vi "Asylum_Driver.vi"() -> ()   [LabVIEW 2019]
uses:
  subVIs/AFM API/AFM_Driver_Manager/AFM_Driver_Manager.PublicEvents.ctl
  subVIs/AFM API/AFM_Driver_Manager/AFM_Driver_Manager.PublicMethods.ctl
  <userlib>/LevyLab/Relay Box/Typedefs/Resistor--enum.ctl
  <userlib>/LevyLab/Configuration/Configuration.lvclass
  Type Defs/Asylum Configuration.ctl
  <vilib>/Utility/sysdir.llb/Get System Directory.vi
  <userlib>/LevyLab/Relay Box/Relay-Box.lvclass
  subVIs/AFM API/AFM_Driver_Manager/AFM_Driver_Manager.lvclass
panel:
  out "Debug Mode?":bool
  in  "Writing Setpoint":dbl caption="Numeric"
  in  "Interpolation (um)":dbl=0.1 caption="Numeric"
  in  "Amplifier":dbl=20.0 caption="Numeric"
  in  "Move Setpoint":dbl caption="Numeric"
  in  "Levylab_Public_Methods_Do_Not_Rename":T1
  in  "Levylab_Public_Events_Do_Not_Rename":T2
  # "Asylum AFM"
  # "Hardware Setup"
  # "Writing Setup"
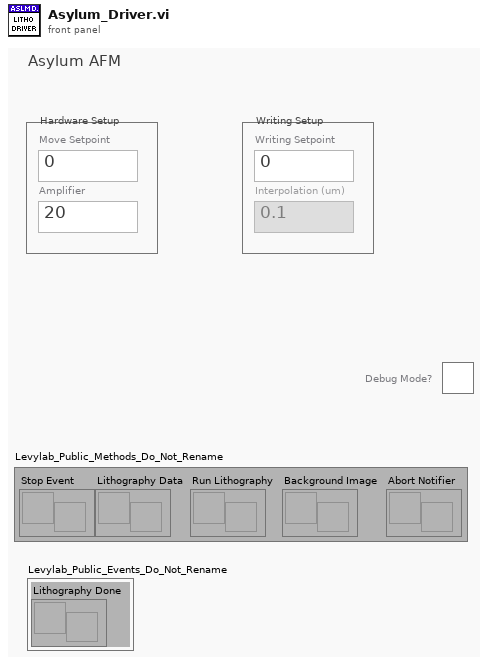
[diagram p1: front panel]
types:
  T1 = typedef "AFM_Driver_Manager.lvclass/AFM_Driver_Manager.PublicMethods.ctl" = cluster{"Stop Event":refnum<user-event>, "Lithography Data":refnum<user-event>, "Run Lithography":refnum<user-event>, "Background Image":refnum<user-event>, "Abort Notifier":refnum<user-event>}
  T2 = typedef "AFM_Driver_Manager.lvclass/AFM_Driver_Manager.PublicEvents.ctl" = cluster{"Lithography Done":refnum<user-event>}
  T3 = enum32{"invalid app kind", "Development System", "Run Time System", "Student Edition", "Embedded LabVIEW", "Evaluation", "Custom"}
  T4 = enum32{"Invalid", "Standard", "Closed", "Hidden", "Minimized", "Maximized"}
  T5 = typedef "Asylum Configuration.ctl" = cluster{"Move Setpoint":dbl, "Amplifier":dbl, "Writing Setpoint":dbl, "Interpolation":dbl, "Debug":bool}
  T6 = typedef "Relay-Box.lvclass/Resistor--enum.ctl" = enum16{"open", "discharge tip", "0 ohms", "100k ohm", "10M ohm", "1G ohm"}
  T7 = cluster{"Core":cluster{"Current VI Reference":refnum<vi>, "Close Panel on Exit?":bool}, "Lithography Data":cluster{"Name":string, "Litho":cluster{"X":dbl, "Y":dbl, "Speed":dbl, "Voltage":dbl}[], "Set Resistance":T6, "Meta":variant}[], "Application":refnum<k7>, "Offsets":cluster{"X":dbl, "Y":dbl}, "Background Image":path, "Writing Setpoint":dbl, "Move Setpoint":dbl, "Interpolation (um)":dbl, "Debug?":bool, "Amplifier":dbl, "Events":T2, "Abort Notifier":refnum<notifier>, "Configuration":refnum<class "Configuration.lvclass">, "Lithography Data (Conv)":cluster{"Name":string, "Litho":cluster{"X":dbl, "Y":dbl, "Speed":dbl, "Voltage":dbl}[], "Set Resistance":T6, "Meta":variant}[]}
  T8 = cluster{"Name":string, "Litho":cluster{"X":dbl, "Y":dbl, "Speed":dbl, "Voltage":dbl}[], "Set Resistance":T6, "Meta":variant}[]
  T9 = cluster{"Current VI Reference":refnum<vi>, "Close Panel on Exit?":bool}
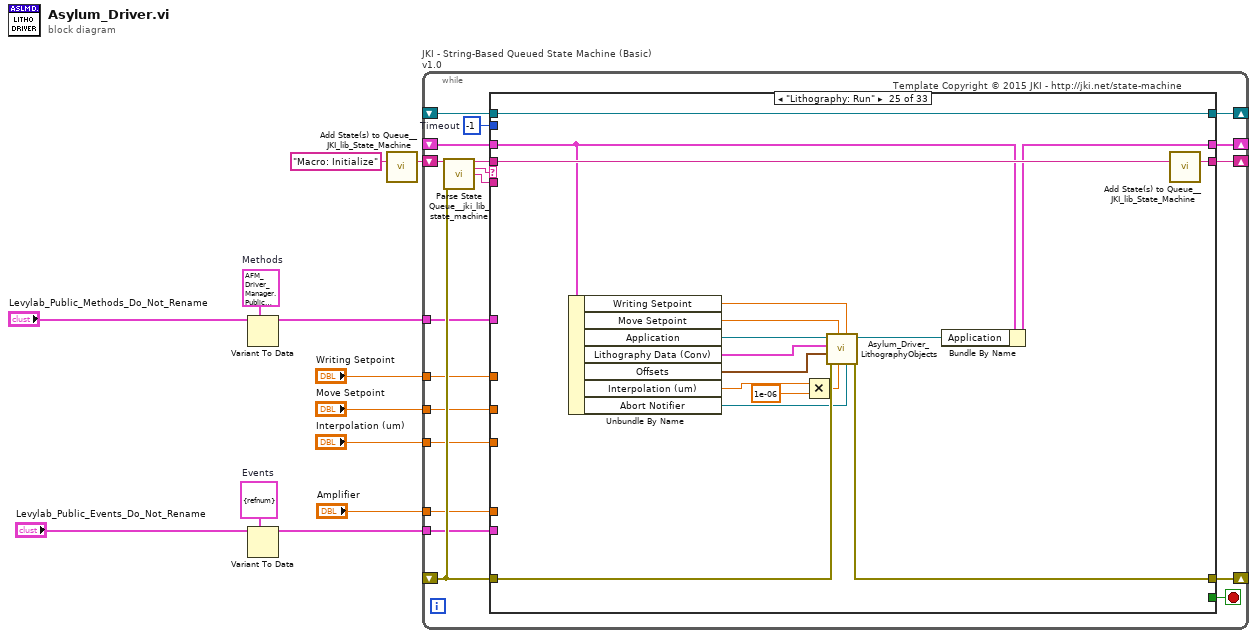
[diagram p0: block diagram]
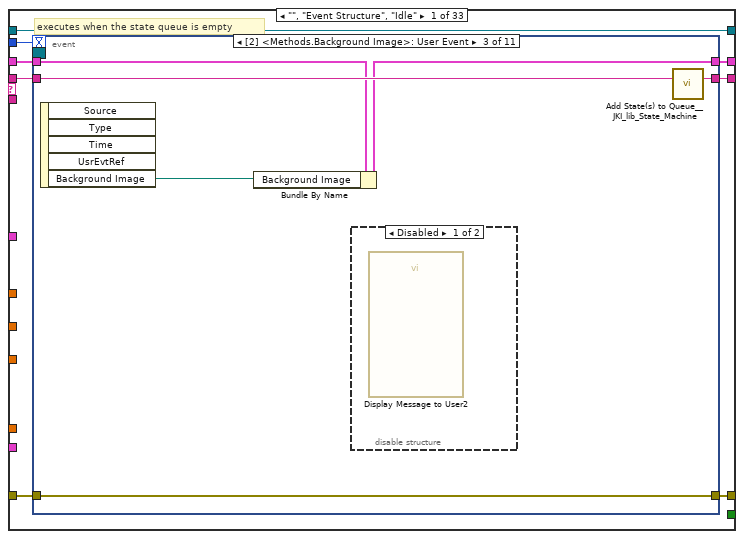
[diagram p2: hidden frame]
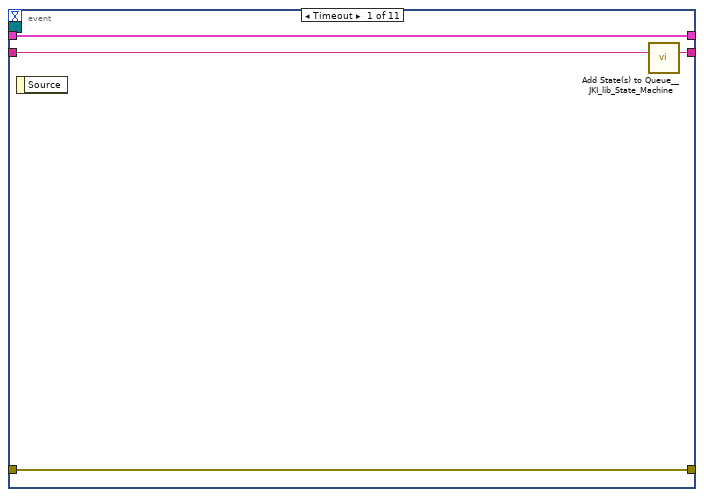
[diagram p3: hidden frame]
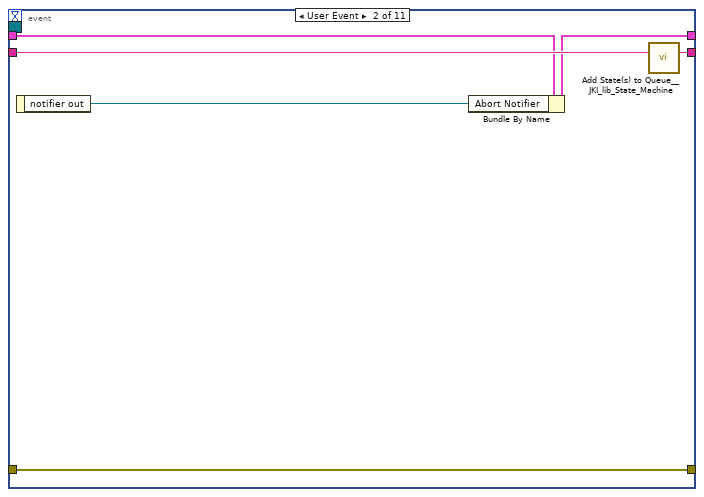
[diagram p4: hidden frame]
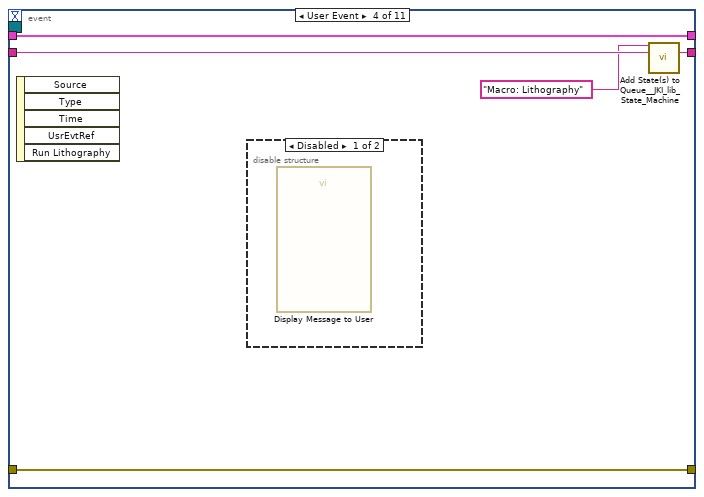
[diagram p6: hidden frame]
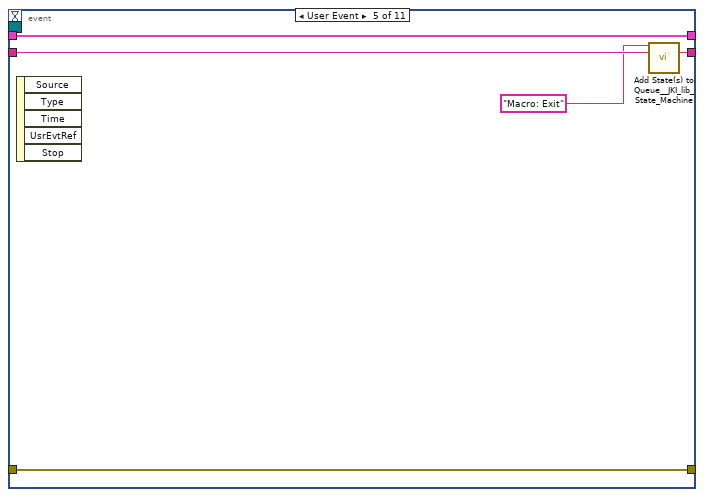
[diagram p8: hidden frame]
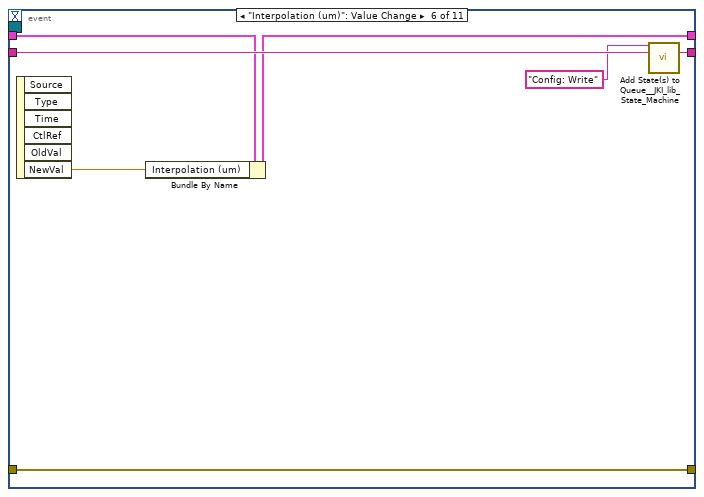
[diagram p9: hidden frame]
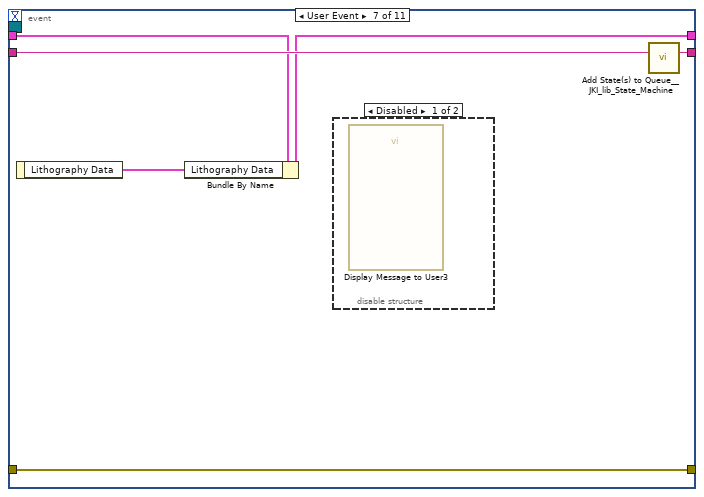
[diagram p10: hidden frame]
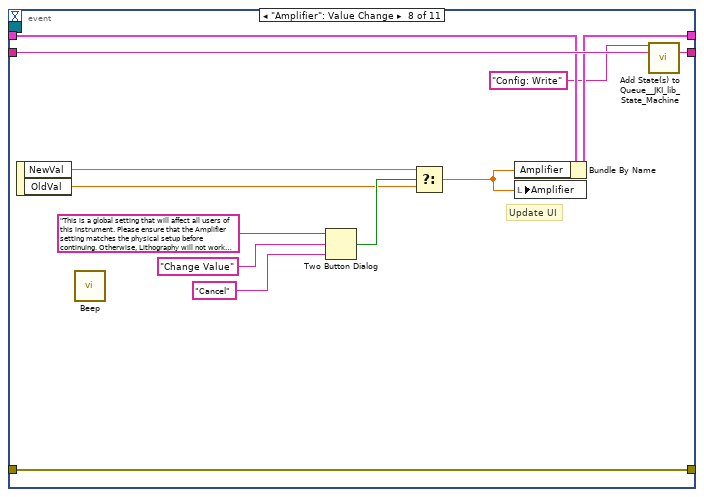
[diagram p12: hidden frame]
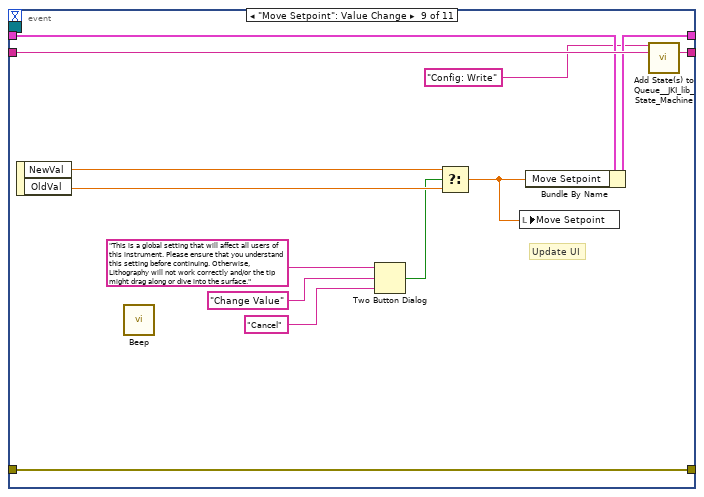
[diagram p13: hidden frame]
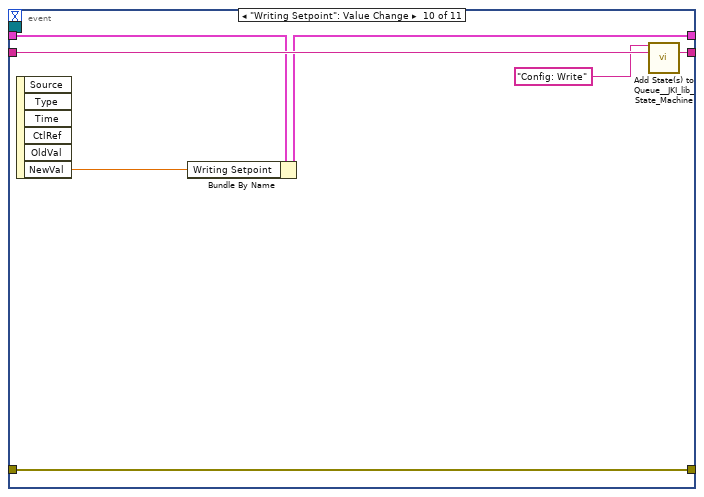
[diagram p14: hidden frame]
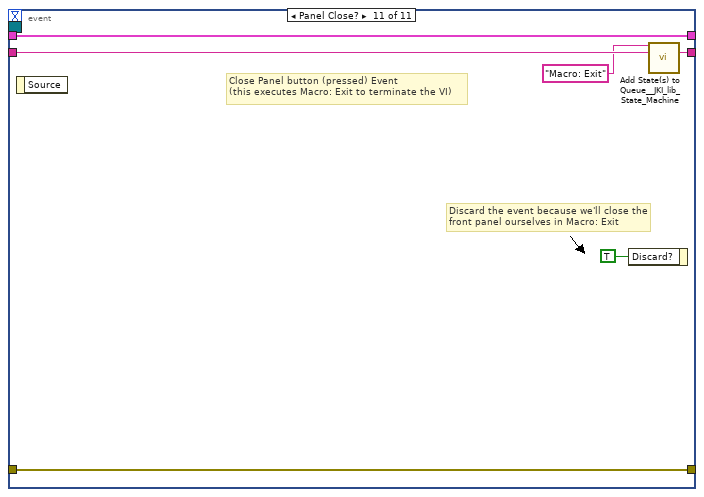
[diagram p15: hidden frame]
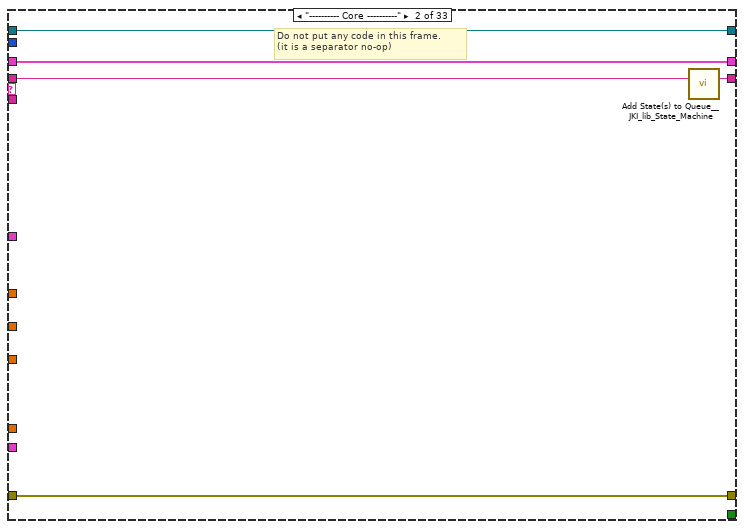
[diagram p16: hidden frame]
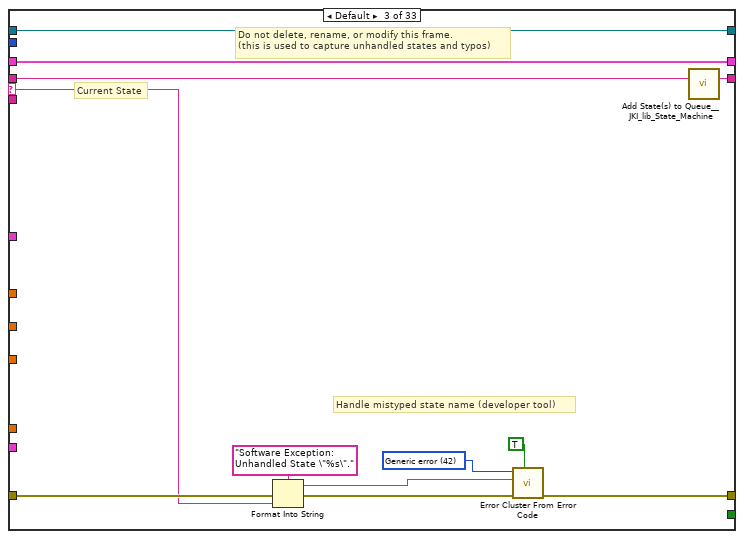
[diagram p17: hidden frame]
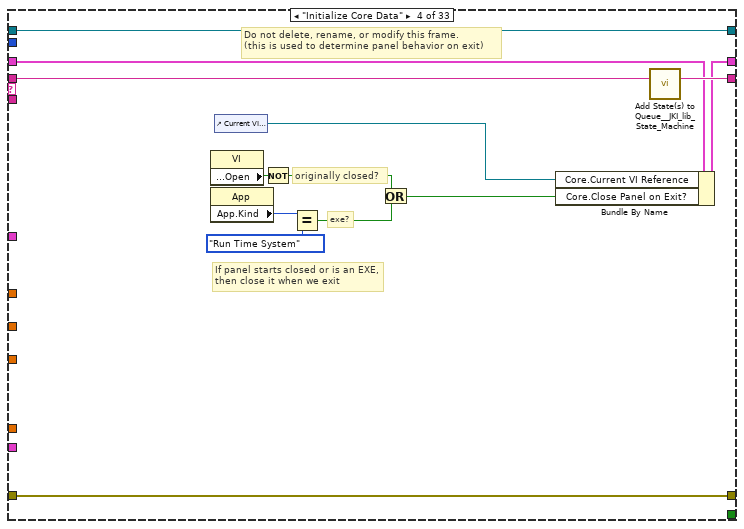
[diagram p18: hidden frame]
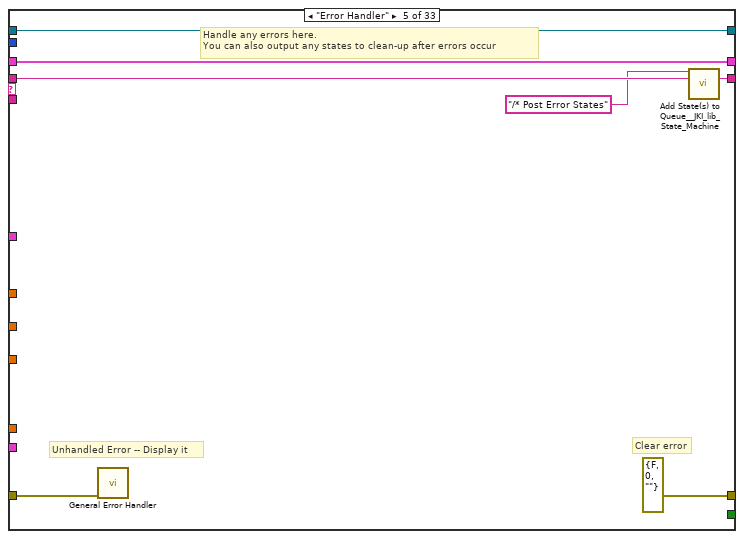
[diagram p19: hidden frame]
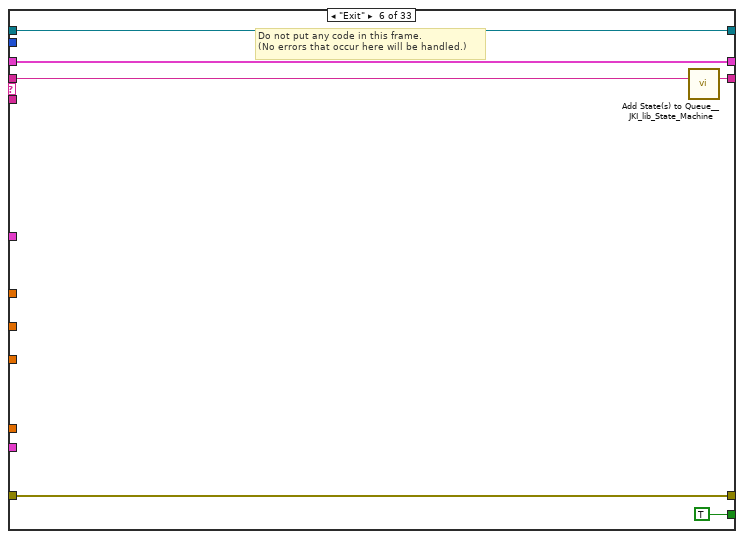
[diagram p20: hidden frame]
diagram:
  w2 = T1 {"Stop Event"=refnum, "Lithography Data"=refnum, "Run Lithography"=refnum, "Background Image"=refnum, "Abort Notifier"=refnum}  # Methods
  w1 = T2 {"Lithography Done"=refnum}  # Events
  n1 = Variant To Data(type=w2, Variant="Levylab_Public_Methods_Do_Not_Rename") -> (data=w6:T1)  [unwired: 1 in, 1 out]
  n2 = Variant To Data(type=w1, Variant="Levylab_Public_Events_Do_Not_Rename") -> (data=w4:T2)  [unwired: 1 in, 1 out]
  n3 = call <vilib>:"Add State(s) to Queue__JKI_lib_State_Machine.vi"("State(s) in (\"\")"="Macro: Initialize") -> ("States Out"=w12:string)  [unwired: 14 in]
  n4 = while "JKI - String-Based Queued State Machine (Basic) v1.0" {
    shift-right: [w23] -> _
    shift-left: _ -> [w22]
    shift-right: [w31] -> _
    shift-left: _ -> [w30]
    shift-right: [w25] -> _
    shift-left: w12 -> [w26]
    tunnel: "Writing Setpoint" -> [w20]
    tunnel: "Move Setpoint" -> [w19]
    tunnel: "Interpolation (um)" -> [w18]
    shift-right: [w17] -> _
    shift-left: _ -> [w16]
    tunnel: w6 -> [w15]
    tunnel: "Amplifier" -> [w14]
    tunnel: w4 -> [w13]
    stop <- w24 stop-if-true
    w21 = -1  # Timeout
    # "Template Copyright © 2015 JKI - http://jki.net/state-machine"
    n5 = call <vilib>:"Parse State Queue__jki_lib_state_machine.vi"("State Queue"=w26, "Error In (no error)"=w30) -> ("Remaining States"=w28:string, "Current State"=w29:string, "Arguments"=w27:string)  [unwired: 11 in]
    n6 = case shown="\"Lithography: Run\"" w29 {
      selector: w29 -> [_ _ w124 _ _ _ _ _ _ _ _ _ _ _ _ _ _ _ _ _ _ _ _ _ _ _ _ _ _ _ _ _ _]
      tunnel: w28 -> [w37 w121 w128 w146 w152 w159 w164 w184 w190 w196 w203 w208 w214 w219 w225 w237 w265 w271 w277 w288 w293 w311 w336 w347 w364 w372 w378 w387 w401 w409 w426 w444 w455]
      tunnel: w27 -> [_ _ _ _ _ _ _ _ _ _ _ _ _ _ w222 w233 _ _ _ _ _ _ w319 _ _ _ _ _ _ _ _ _ _]
      tunnel: w22 -> [w35 w119 w126 w138 w150 w157 w162 _ w187 w194 w199 w206 w212 w216 w223 w235 w263 w269 w275 w286 w291 w307 w329 w343 w351 w369 w376 w382 w396 w405 w422 w440 w451]
      tunnel: [w39 w122 w133 w147 errorcluster {"status"=FALSE, "code"=0, "source"=""} ("error out") w160 w165 w185 w191 w197 w204 w209 w215 w220 w226 w238 w266 w272 w278 w289 w294 w299 w333 w348 w365 w374 w379 w388 w403 w410 w413 w434 w446] -> w31
      tunnel: w30 -> [w38 w122 w132 w147 w153 w160 w165 w185 w192 w197 w198 w210 w215 w220 w227 w239 w266 w272 w278 w289 w294 w300 w332 w349 w366 w373 w379 w390 w402 w410 w412 w433 w445]
      tunnel: [w36 w120 w127 w145 w151 w158 w163 w183 w189 w195 w202 w207 w213 w218 w224 w236 w264 w270 w276 w287 w292 w310 w335 w346 w363 w371 w377 w386 w400 w408 w425 w443 w454] -> w25
      tunnel: [_ _ _ _ _ TRUE _ _ _ _ _ _ _ _ _ _ _ _ _ _ _ _ _ _ _ _ _ _ _ _ _ _ _] -> w24
      tunnel: [w34 w119 w126 w144 w150 w157 w162 w182 w187 w194 w199 w206 w212 w216 w223 w235 w263 w269 w275 w286 w291 w308 w331 w342 w352 w369 w376 w383 w398 w406 w423 w441 w452] -> w23
      tunnel: w21 -> [w33 _ _ _ _ _ _ _ _ _ _ _ _ _ _ _ _ _ _ _ _ _ _ _ _ _ _ _ _ _ _ _ _]
      tunnel: w20 -> [_ _ _ _ _ _ _ w177 _ _ _ _ _ _ _ _ _ _ _ _ _ _ _ _ _ _ _ _ _ _ _ _ _]
      tunnel: w19 -> [_ _ _ _ _ _ _ w176 _ _ _ _ _ _ _ _ _ _ _ _ _ _ _ _ _ _ _ _ _ _ _ _ _]
      tunnel: w18 -> [_ _ _ _ _ _ _ w167 _ _ _ _ _ _ _ _ _ _ _ _ _ _ _ _ _ _ _ _ _ _ _ _ _]
      tunnel: [w32 w118 w123 w135 w148 w155 w161 w175 w186 w193 w201 w205 w211 w217 w221 w232 w262 w268 w273 w279 w290 w309 w334 w341 w360 w370 w375 w385 w399 w407 w424 w442 w453] -> w17
      tunnel: w16 -> [w32 w118 w123 w135 w148 w155 w161 w175 w186 w193 _ w205 w211 w217 w221 w232 w262 w268 w273 w279 w290 w309 w334 w341 w360 w370 w375 w385 w399 w407 w424 w442 w453]
      tunnel: w15 -> [_ _ _ _ _ _ _ _ _ _ w200 _ _ _ _ _ _ _ _ _ _ _ _ _ _ _ _ _ _ _ _ _ _]
      tunnel: w14 -> [_ _ _ _ _ _ _ w174 _ _ _ _ _ _ _ _ _ _ _ _ _ _ _ _ _ _ _ _ _ _ _ _ _]
      tunnel: w13 -> [_ _ _ _ _ _ _ w173 _ _ _ _ _ _ _ _ _ _ _ _ _ _ _ _ _ _ _ _ _ _ _ _ _]
      frame "", "Event Structure", "Idle" {
        # "executes when the state queue is empty"
        n7 = event shown="[2] <Methods.Background Image>: User Event" {
          selector: w32 -> [_ _ _ _ _ _ _ _ _ _ _]
          dyn-events: _ -> [_ _ _ _ _ _ _ _ _ _ _]
          timeout: w33 -> [_ _ _ _ _ _ _ _ _ _ _]
          tunnel: w37 -> [w42 w48 w54 w59 w64 w71 w77 w90 w103 w110 w116]
          tunnel: [w41 w47 w53 w58 w63 w70 w76 w89 w102 w109 w115] -> w36
          tunnel: w35 -> [w40 w45 w51 w57 w62 w68 w74 w87 w100 w107 w114]
          tunnel: [w43 w49 w55 w60 w65 w72 w78 w91 w104 w111 w117] -> w39
          tunnel: w38 -> [w43 w49 w55 w60 w65 w72 w78 w91 w104 w111 w117]
          tunnel: [w40 w46 w52 w57 w62 w69 w75 w88 w101 w108 w114] -> w34
          event Timeout {
            n8 = event-data() -> ()  [unwired: 1 in, 1 out]
            n9 = call <vilib>:"Add State(s) to Queue__JKI_lib_State_Machine.vi"("State(s) in (\"\")"=w42) -> ("States Out"=w41:string)  [unwired: 14 in]
          }
          event User Event {
            n10 = event-data() -> ("notifier out"=w44:refnum<notifier>)  [unwired: 1 in]
            n11 = Bundle By Name(cluster=w45, "Abort Notifier"=w44) -> (w46:T7)
            n12 = call <vilib>:"Add State(s) to Queue__JKI_lib_State_Machine.vi"("State(s) in (\"\")"=w48) -> ("States Out"=w47:string)  [unwired: 14 in]
          }
          event User Event {
            n13 = event-data() -> ("Background Image"=w50:path)  [unwired: 1 in, 4 out]
            n14 = Bundle By Name(cluster=w51, "Background Image"=w50) -> (w52:T7)
            n15 = disable-structure shown="Disabled" {
              frame Disabled {
                n16 = call "Display Message to User2"() -> ()  [unwired: 10 in, 2 out]
              }
              frame Enabled {
              }
            }
            n17 = call <vilib>:"Add State(s) to Queue__JKI_lib_State_Machine.vi"("State(s) in (\"\")"=w54) -> ("States Out"=w53:string)  [unwired: 14 in]
          }
          event User Event {
            n18 = event-data() -> ()  [unwired: 1 in, 5 out]
            n19 = disable-structure shown="Disabled" {
              frame Disabled {
                n20 = call "Display Message to User"() -> ()  [unwired: 10 in, 2 out]
              }
              frame Enabled {
              }
            }
            n21 = call <vilib>:"Add State(s) to Queue__JKI_lib_State_Machine.vi"("State(s) in Front (\"\")"="Macro: Lithography" ("State(s) in Front (\"\")"), "State(s) in (\"\")"=w59) -> ("States Out"=w58:string)  [unwired: 13 in]
          }
          event User Event {
            n22 = event-data() -> ()  [unwired: 1 in, 5 out]
            n23 = call <vilib>:"Add State(s) to Queue__JKI_lib_State_Machine.vi"("State(s) in Front (\"\")"="Macro: Exit", "State(s) in (\"\")"=w64) -> ("States Out"=w63:string)  [unwired: 13 in]
          }
          event "Interpolation (um)": Value Change {
            n24 = event-data() -> ("NewVal"=w66:dbl)  [unwired: 1 in, 5 out]
            n25 = Bundle By Name(cluster=w68, "Interpolation (um)"=w66) -> (w69:T7)
            n26 = call <vilib>:"Add State(s) to Queue__JKI_lib_State_Machine.vi"("State(s) in Front (\"\")"="Config: Write" ("State(s) in Front (\"\")"), "State(s) in (\"\")"=w71) -> ("States Out"=w70:string)  [unwired: 13 in]
          }
          event User Event {
            n27 = event-data() -> ("Lithography Data"=w73:T8)  [unwired: 1 in]
            n28 = Bundle By Name(cluster=w74, "Lithography Data"=w73) -> (w75:T7)
            n29 = disable-structure shown="Disabled" {
              frame Disabled {
                n30 = call "Display Message to User3"() -> ()  [unwired: 10 in, 2 out]
              }
              frame Enabled {
              }
            }
            n31 = call <vilib>:"Add State(s) to Queue__JKI_lib_State_Machine.vi"("State(s) in (\"\")"=w77) -> ("States Out"=w76:string)  [unwired: 14 in]
          }
          event "Amplifier": Value Change {
            # "Update UI"
            n32 = event-data() -> ("NewVal"=w85:dbl, "OldVal"=w83:dbl)  [unwired: 1 in]
            n33 = call <vilib>:"Beep.vi"() -> ()  [unwired: 12 in]
            n34 = Two Button Dialog(message="This is a global setting that will affect all users of this instrument. Please ensure that the Amplifier setting matches the physical setup before continuing. Otherwise, Lithography will not work correctly.", 1:"Cancel" ("F button name (\"Cancel\")"), 2:"Change Value" ("T button name (\"OK\")")) -> (T button?=w84:bool)
            n35 = Select(t=w85, s=w84, f=w83) -> (s? t:f=w82:dbl)
            n36 = Bundle By Name(cluster=w87, "Amplifier"=w82) -> (w88:T7)
            n37 = local write "Amplifier"(w82) -> ()
            n38 = call <vilib>:"Add State(s) to Queue__JKI_lib_State_Machine.vi"("State(s) in Front (\"\")"="Config: Write" ("State(s) in Front (\"\")"), "State(s) in (\"\")"=w90) -> ("States Out"=w89:string)  [unwired: 13 in]
          }
          event "Move Setpoint": Value Change {
            # "Update UI"
            n39 = event-data() -> ("NewVal"=w96:dbl, "OldVal"=w97:dbl)  [unwired: 1 in]
            n40 = call <vilib>:"Beep.vi"() -> ()  [unwired: 12 in]
            n41 = Two Button Dialog(message="This is a global setting that will affect all users of this instrument. Please ensure that you understand this setting before continuing. Otherwise, Lithography will not work correctly and/or the tip might drag along or dive into the surface.", 1:"Cancel" ("F button name (\"Cancel\")"), 2:"Change Value" ("T button name (\"OK\")")) -> (T button?=w95:bool)
            n42 = Select(t=w96, s=w95, f=w97) -> (s? t:f=w93:dbl)
            n43 = local write "Move Setpoint"(w93) -> ()
            n44 = Bundle By Name(cluster=w100, "Move Setpoint"=w93) -> (w101:T7)
            n45 = call <vilib>:"Add State(s) to Queue__JKI_lib_State_Machine.vi"("State(s) in Front (\"\")"="Config: Write" ("State(s) in Front (\"\")"), "State(s) in (\"\")"=w103) -> ("States Out"=w102:string)  [unwired: 13 in]
          }
          event "Writing Setpoint": Value Change {
            n46 = event-data() -> ("NewVal"=w106:dbl)  [unwired: 1 in, 5 out]
            n47 = Bundle By Name(cluster=w107, "Writing Setpoint"=w106) -> (w108:T7)
            n48 = call <vilib>:"Add State(s) to Queue__JKI_lib_State_Machine.vi"("State(s) in Front (\"\")"="Config: Write" ("State(s) in Front (\"\")"), "State(s) in (\"\")"=w110) -> ("States Out"=w109:string)  [unwired: 13 in]
          }
          event Panel Close? {
            # "Discard the event because we'll close the front panel ourselves in Macro: Exit"
            # "Close Panel button (pressed) Event\n(this executes Macro: Exit to terminate the VI)"
            n49 = event-data() -> ()  [unwired: 1 in, 1 out]
            n50 = event-data("Discard?"=TRUE) -> ()  [unwired: 1 in, 1 out]
            n51 = call <vilib>:"Add State(s) to Queue__JKI_lib_State_Machine.vi"("State(s) in Front (\"\")"="Macro: Exit", "State(s) in (\"\")"=w116) -> ("States Out"=w115:string)  [unwired: 13 in]
          }
        }
      }
      frame "---------- Core ----------" {
        # "Do not put any code in this frame.\n(it is a separator no-op)"
        n52 = call <vilib>:"Add State(s) to Queue__JKI_lib_State_Machine.vi"("State(s) in (\"\")"=w121) -> ("States Out"=w120:string)  [unwired: 14 in]
      }
      frame Default {
        w130 = 42 items=["No error", "Argument error", "Memory is full", "Out of zone", "End of file", "File already open", "Generic file I/O error", "File not found", "File permission error", "Disk is full", "Duplicate path", "Too many files open", "System feature not enabled", "Resource file not found", "Cannot add resource", "Resource not found", "Image not found", "Image memory error", "Pen does not exist", "Config type invalid", "Config token not found", "Config parse error", "Config memory error", "Bad external code format", "Bad external code offset", "External code not present", "Null window", "Destroy window error", "Null menu", "Print aborted", "Bad print record", "Print driver error", "Windows error during printing", "Memory error during printing", "Print dialog error", "Generic print error", "Invalid device refnum", "Device not found", "Device parameter error", "Device unit error", "Cannot open device", "Device call aborted", "Generic error", "Cancelled by user", "Object ID too low", "Object ID too high", "Object not in heap", "Unknown heap", "Unknown object (invalid DefProc)", "Unknown object (DefProc not in table)", "Message out of range", "Invalid (null) method", "Unknown message", "Manager call not supported", "Bad address", "Network operation in progress", "Network operation timed out", "Connection is busy", "Network attribute not supported", "Network error", "Address in use", "System out of memory", "Connection aborted", "Connection refused", "Not connected", "Already connected", "Connection closed", "Initialization error (interapplication manager)", "Bad occurrence", "Wait on unbound occurrence handler", "Occurrence queue overflow", "Datalog type conflict", "Unused", "Unrecognized type (interapplication manager)", "Memory corrupt", "Failed to make temporary DLL", "Old CIN version", "Drag socket not found", "Failed to load drop-object", "Failed to register OLE object", "Failed to release OLE object", "Format specifier type mismatch", "Unknown format specifier", "Too few format specifiers", "Too many format specifiers", "Scan failed", "Newer CIN version", "Error converting to variant", "Runtime menu error", "Password tampered", "Variant attribute not found", "Incompatible variant data type", "Event data is not available", "Event Store is not present", "Occurrence is not found", "Event Queue is not created", "Event info is not available", "Refnum passed is NULL", "Error retrieving Class GUID", "Error retrieving CoClass GUID", "Error retrieving TypeLib GUID.", "Bad built application magic bytes.", "Specific driver is different from the specific driver associated with the Logical Name.", "There is no session opened to the class driver.", "Max Error", "MAX - Error with config objects", "MAX - Error loading configuration", "MAX - Group not supported"]
        # "Current State"
        # "Do not delete, rename, or modify this frame.\n(this is used to capture unhandled states and typos)"
        # "Handle mistyped state name (developer tool)"
        n53 = Format Into String(format string="Software Exception: Unhandled State \"%s\"." ("message"), error in=w132, w124) -> (resulting string=w129:string, error out=w134:errorcluster)  [unwired: 1 in]
        n54 = call <vilib>:"Error Cluster From Error Code.vi"("show call chain? (False)"=TRUE, "error in (no error)"=w134, "error message (\"\")"=w129, "error code (0)"=w130) -> ("error out"=w133:errorcluster)  [unwired: 5 in]
        n55 = call <vilib>:"Add State(s) to Queue__JKI_lib_State_Machine.vi"("State(s) in (\"\")"=w128) -> ("States Out"=w127:string)  [unwired: 14 in]
      }
      frame "Initialize Core Data" {
        # "Do not delete, rename, or modify this frame.\n(this is used to determine panel behavior on exit)"
        # "originally closed?"
        # "exe?"
        # "If panel starts closed or is an EXE, then close it when we exit"
        n56 = property class="VI"() -> ("Front Panel.Open"=w143:bool)  [unwired: 2 in, 2 out]
        n57 = property class="App"() -> ("App.Kind"=w142:T3)  [unwired: 2 in, 2 out]
        n58 = control-ref of="Current VI Reference"() -> (w136:refnum<vi>)
        n59 = Not(x=w143) -> (.not. x?=w140:bool)
        n60 = Equal?(x=w142, y=T3."Run Time System" ("Application:Kind")) -> (x = y?=w139:bool)
        n61 = Or(x=w140, y=w139) -> (x .or. y?=w137:bool)
        n62 = Bundle By Name(cluster=w138, "Core.Current VI Reference"=w136, "Core.Close Panel on Exit?"=w137) -> (w144:T7)
        n63 = call <vilib>:"Add State(s) to Queue__JKI_lib_State_Machine.vi"("State(s) in (\"\")"=w146) -> ("States Out"=w145:string)  [unwired: 14 in]
      }
      frame "Error Handler" {
        # "Unhandled Error -- Display it"
        # "Handle any errors here.\nYou can also output any states to clean-up after errors occur"
        # "Clear error"
        n64 = call <vilib>:"General Error Handler.vi"("error in (no error)"=w153) -> ()  [unwired: 10 in, 5 out]
        n65 = call <vilib>:"Add State(s) to Queue__JKI_lib_State_Machine.vi"("State(s) in Front (\"\")"="/* Post Error States", "State(s) in (\"\")"=w152) -> ("States Out"=w151:string)  [unwired: 13 in]
      }
      frame "Exit" {
        # "Do not put any code in this frame.\n(No errors that occur here will be handled.)"
        n66 = call <vilib>:"Add State(s) to Queue__JKI_lib_State_Machine.vi"("State(s) in (\"\")"=w159) -> ("States Out"=w158:string)  [unwired: 14 in]
      }
      frame "---------- Data ----------" {
        # "Do not put any code in this frame.\n(It is a separator no-op. You can make a copy of this frame to create a new Data frame)"
        n67 = call <vilib>:"Add State(s) to Queue__JKI_lib_State_Machine.vi"("State(s) in (\"\")"=w164) -> ("States Out"=w163:string)  [unwired: 14 in]
      }
      frame "Data: Initialize" {
        w166 = T8 []  # Lithography Data (Conv)
        w169 = T8 []  # Lithography Data
        w170 = TRUE  # Debug?
        w171 = refnum<class "Configuration.lvclass"> refnum  # Configuration
        w172 = refnum<notifier> refnum  # Abort Notifier
        w178 = path ""  # Background Image
        w179 = cluster{"X":dbl, "Y":dbl} {"X"=0.0, "Y"=0.0}  # Offsets
        w180 = refnum<k7> refnum  # Application
        w181 = T9 {"Current VI Reference"=refnum, "Close Panel on Exit?"=FALSE}  # Core
        # "Initialize the shift-register data, here.\n(data names are defined by what you wire into the bundle function)"
        n68 = Multiply(x=w167, y=1e-06) -> ()  [unwired: 1 out]
        n69 = Bundle("Core"=w181, "Lithography Data"=w169, "Application"=w180, "Offsets"=w179, "Background Image"=w178, "Writing Setpoint"=w177, "Move Setpoint"=w176, "Interpolation (um)"=w167, "Debug?"=w170, "Amplifier"=w174, "Events"=w173, "Abort Notifier"=w172, "Configuration"=w171, "Lithography Data (Conv)"=w166) -> (w182:T7)  [unwired: 1 in]
        n70 = call <vilib>:"Add State(s) to Queue__JKI_lib_State_Machine.vi"("State(s) in (\"\")"=w184) -> ("States Out"=w183:string)  [unwired: 14 in]
      }
      frame "Data: Cleanup" {
        # "Cleanup any data and references, here.\n(this is called automatically, by the Macro: Exit)"
        n71 = Unbundle By Name(w187) -> ("Core.Current VI Reference"=w188:refnum<vi>)
        n72 = Close Reference(reference=w188, error in (no error)=w192) -> (error out=w191:errorcluster)
        n73 = call <vilib>:"Add State(s) to Queue__JKI_lib_State_Machine.vi"("State(s) in (\"\")"=w190) -> ("States Out"=w189:string)  [unwired: 14 in]
      }
      frame "---------- Events ----------" {
        # "Do not put any code in this frame.\n(It is a separator no-op. You can make a copy of this frame to create a new UI frame)"
        n74 = call <vilib>:"Add State(s) to Queue__JKI_lib_State_Machine.vi"("State(s) in (\"\")"=w196) -> ("States Out"=w195:string)  [unwired: 14 in]
      }
      frame "Events: Register" {
        # "Do not put any code in this frame.\n(It is a separator no-op. You can make a copy of this frame to create a new UI frame)"
        n75 = register-events(error in=w198, w200) -> (reference out=w201:refnum<event-registration>, error out=w204:errorcluster)  [unwired: 1 in]
        n76 = call <vilib>:"Add State(s) to Queue__JKI_lib_State_Machine.vi"("State(s) in (\"\")"=w203) -> ("States Out"=w202:string)  [unwired: 14 in]
      }
      frame "Events: Unregister" {
        # "Do not put any code in this frame.\n(It is a separator no-op. You can make a copy of this frame to create a new UI frame)"
        n77 = Unregister For Events(event registration refnum=w205, error in=w210) -> (error out=w209:errorcluster)
        n78 = call <vilib>:"Add State(s) to Queue__JKI_lib_State_Machine.vi"("State(s) in (\"\")"=w208) -> ("States Out"=w207:string)  [unwired: 14 in]
      }
      frame "---------- UI ----------" {
        # "Do not put any code in this frame.\n(It is a separator no-op. You can make a copy of this frame to create a new UI frame)"
        n79 = call <vilib>:"Add State(s) to Queue__JKI_lib_State_Machine.vi"("State(s) in (\"\")"=w214) -> ("States Out"=w213:string)  [unwired: 14 in]
      }
      frame "UI: Initialize" {
        # "Initialize the User Interface, here.\n(this is called automatically, by the Macro: Init)"
        n80 = call <vilib>:"Add State(s) to Queue__JKI_lib_State_Machine.vi"("State(s) in (\"\")"=w219) -> ("States Out"=w218:string)  [unwired: 14 in]
      }
      frame "UI: Cursor Set" {
        # "Argument"
        # "Set and Unset Cursor Busy.\n(Usage: \"UI: Cursor Set >> Busy|Idle\")"
        n81 = case shown="\"Idle\", Default" w222 {
          tunnel: w227 -> [w229 w231]
          tunnel: [w228 w230] -> w226
          frame "Idle", Default {
            n82 = call <vilib>:"Unset Busy.vi"("error in (no error)"=w229) -> ("error out"=w228:errorcluster)  [unwired: 10 in]
          }
          frame "Busy" {
            n83 = call <vilib>:"Set Busy.vi"("error in (no error)"=w231) -> ("error out"=w230:errorcluster)  [unwired: 9 in, 1 out]
          }
        }
        n84 = call <vilib>:"Add State(s) to Queue__JKI_lib_State_Machine.vi"("State(s) in (\"\")"=w225) -> ("States Out"=w224:string)  [unwired: 14 in]
      }
      frame "UI: Front Panel State" {
        # "Argument"
        # "Set Front Panel Open or Closed\n(Usage: \"UI: Front Panel State >> Open|Close\")"
        n85 = Unbundle By Name(w235) -> ("Core.Current VI Reference"=w234:refnum<vi>)
        n86 = case shown="\"Open\", Default" w233 {
          tunnel: w239 -> [w244 w256]
          tunnel: [w245 w257] -> w238
          tunnel: w234 -> [w242 w254]
          frame "Open", Default {
            n87 = property class="VI"(reference=w242, error in=w244) -> (reference out=w241:refnum<vi>, error out=w243:errorcluster, "Front Panel.Open"=w240:bool)
            n88 = case shown="False" w240 {
              tunnel: [w250 w251] -> w245
              tunnel: w243 -> [w249 w251]
              tunnel: w241 -> [w246 _]
              frame False {
                n89 = invoke class="VI" method="FP.Open"(reference=w246, error in=w249, "Activate"=TRUE, "State"=T4."Standard") -> (error out=w250:errorcluster)  [unwired: 1 in, 4 out]
              }
              frame True {
              }
            }
          }
          frame "Close" {
            n90 = property class="VI"(reference=w254, error in=w256) -> (reference out=w253:refnum<vi>, error out=w255:errorcluster, "Front Panel.Open"=w252:bool)
            n91 = case shown="True" w252 {
              tunnel: [w258 w261] -> w257
              tunnel: w255 -> [w258 w260]
              tunnel: w253 -> [_ w259]
              frame False {
              }
              frame True {
                n92 = invoke class="VI" method="FP.Close"(reference=w259, error in=w260) -> (error out=w261:errorcluster)  [unwired: 1 in, 2 out]
              }
            }
          }
        }
        n93 = call <vilib>:"Add State(s) to Queue__JKI_lib_State_Machine.vi"("State(s) in (\"\")"=w237) -> ("States Out"=w236:string)  [unwired: 14 in]
      }
      frame "---------- Macro ----------" {
        # "Do not put any code in this frame.\n(It is a separator no-op. You can make a copy of this frame to create a new Macro frame)"
        n94 = call <vilib>:"Add State(s) to Queue__JKI_lib_State_Machine.vi"("State(s) in (\"\")"=w265) -> ("States Out"=w264:string)  [unwired: 14 in]
      }
      frame "Macro: Lithography" {
        # "Do not put any code in this frame.\n(It is a separator no-op. You can make a copy of this frame to create a new Macro frame)"
        n95 = call <vilib>:"Add State(s) to Queue__JKI_lib_State_Machine.vi"("State(s) in Front (\"\")"="Asylum: Open Reference\nLithography: Check Mode\nLithography: Init\nLithography: Show Spot >> TRUE\nLithography: Run\nLithography: Show Spot >> FALSE\nLithography: Cleanup //must call this state when done\nAsylum: Close Reference", "State(s) in (\"\")"=w271) -> ("States Out"=w270:string)  [unwired: 13 in]
      }
      frame "Macro: Initialize" {
        # "Initialization Macro\n(This is called once, when the VI starts)"
        n96 = call <vilib>:"Add State(s) to Queue__JKI_lib_State_Machine.vi"("State(s) in Front (\"\")"="Data: Initialize\nInitialize Core Data\nEvents: Register\nConfig: Initialize\nConfig: Read\nUI: Initialize\n//Asylum: Open Reference\n//UI: Front Panel State >> Open", "State(s) in (\"\")"=w277) -> ("States Out"=w276:string)  [unwired: 13 in]
      }
      frame "Macro: Exit" {
        # "Exit Macro\n(This is called once, when the VI exits)"
        n97 = Unbundle By Name(w286) -> ("Core.Close Panel on Exit?"=w285:bool)
        n98 = Select(t="UI: Front Panel State >> Close", s=w285, f="") -> (s? t:f=w282:string)
        n99 = call <vilib>:"Add State(s) to Queue__JKI_lib_State_Machine.vi"("State(s) in (\"\")"=w282, "State(s) at Back (\"\")"="//Asylum: Close Reference\nData: Cleanup\nEvents: Unregister\nExit") -> ("States Out"=w280:string)  [unwired: 13 in]
        n100 = call <vilib>:"Add State(s) to Queue__JKI_lib_State_Machine.vi"("State(s) in Front (\"\")"=w280, "State(s) in (\"\")"=w288) -> ("States Out"=w287:string)  [unwired: 13 in]
      }
      frame "---------- Lithography ----------" {
        n101 = call <vilib>:"Add State(s) to Queue__JKI_lib_State_Machine.vi"("State(s) in (\"\")"=w293) -> ("States Out"=w292:string)  [unwired: 14 in]
      }
      frame "Lithography: Check Mode" {
        # "Lithography: Check Mode\nSince the setpoints are opposite in AC and Contact modes, trying to set a negative or small value in AC mode will drive the tip into the surface.  AC mode is fraction of 1 V amplitude (ie 0-1 V), where the lower the value the more force. Contact mode is the deflection, so the lower the value, the lower the force."
        n102 = Unbundle By Name(w307) -> ("Application"=w306:refnum<k7>, "Abort Notifier"=w302:refnum<notifier>)
        n103 = call "Asylum_Driver_GetImagingMode.vi"("error in (no error)"=w300, "Application In"=w306) -> ("error out"=w301:errorcluster, "Imaging Mode"=w304:string, "Application Out"=w305:refnum<k7>)  [unwired: 7 in]
        n104 = call <userlib>:"DebugModeSingleton.vi"("Write?"=FALSE) -> ("Debug Mode?"=w296:bool)  [unwired: 10 in]
        n105 = Equal?(x=w304, y="Contact") -> (x = y?=w297:bool)
        n106 = Or(x=w297, y=w296) -> (x .or. y?=w295:bool)
        n107 = case shown="False" w295 {
          tunnel: w302 -> [w313 _]
          tunnel: w301 -> [w316 w317]
          tunnel: [w312 w317] -> w299
          frame False {
            # "Abort the lithography process to prevent damage"
            # "AFM is not in Contact Mode"
            n108 = call "Display Message to User4"("error in (no error)"=w316) -> ("error out"=w315:errorcluster)  [unwired: 9 in, 1 out]
            n109 = Send Notification(notification=TRUE, notifier=w313, error in (no error)=w315) -> (error out=w312:errorcluster)  [unwired: 1 out]
          }
          frame True {
            # "AFM is in Contact Mode"
          }
        }
        n110 = Bundle By Name(cluster=w307, "Application"=w305) -> (w308:T7)
        n111 = call <vilib>:"Add State(s) to Queue__JKI_lib_State_Machine.vi"("State(s) in (\"\")"=w311) -> ("States Out"=w310:string)  [unwired: 14 in]
      }
      frame "Lithography: Show Spot" {
        n112 = To Upper Case(1:w319) -> (0:w320:string)
        n113 = Match True/False String(2:"FALSE" ("false string"), 3:"TRUE" ("true string"), 4:w320) -> (0:w323:bool)  [unwired: 1 out]
        n114 = Boolean To (0,1)(Boolean=w323) -> (0, 1=w322:i16)
        n115 = Number To Decimal String(number=w322) -> (decimal integer string=w321:string)  [unwired: 1 in]
        n116 = Concatenate Strings("ARExecuteControl(\"ShowXYSpotCheck_1\", \"MasterPanel\", " ("parameterName"), w321, ", \"\")" ("string")) -> (w318:string)
        n117 = Unbundle By Name(w329) -> ("Application"=w328:refnum<k7>)
        n118 = call <userlib>:"Igor_SendCommand.vi"("error in (no error)"=w332, "command"=w318, "Application In"=w328) -> ("error out"=w333:errorcluster, "Application Out"=w330:refnum<k7>)  [unwired: 5 in, 2 out]
        n119 = Bundle By Name(cluster=w329, "Application"=w330) -> (w331:T7)
        n120 = call <vilib>:"Add State(s) to Queue__JKI_lib_State_Machine.vi"("State(s) in (\"\")"=w336) -> ("States Out"=w335:string)  [unwired: 14 in]
      }
      frame "Lithography: Init" {
        n121 = Unbundle By Name(w343) -> ("Background Image"=w338:path, "Lithography Data"=w339:T8, "Amplifier"=w340:dbl)
        n122 = call "Asylum_Driver_LithographyInitialize.vi"("error in (no error)"=w349, "Background Image"=w338) -> ("error out"=w337:errorcluster, "Offset out"=w344:cluster{"X":dbl, "Y":dbl})  [unwired: 8 in]
        n123 = call "Asylum_Driver_Lithography_Convert_Units.vi"("Amplifier"=w340, "error in (no error)"=w337, "Lithography Data"=w339) -> ("error out"=w348:errorcluster, "Lithography Data"=w345:T8)  [unwired: 7 in]
        n124 = Bundle By Name(cluster=w343, "Offsets"=w344, "Lithography Data (Conv)"=w345) -> (w342:T7)
        n125 = call <vilib>:"Add State(s) to Queue__JKI_lib_State_Machine.vi"("State(s) in (\"\")"=w347) -> ("States Out"=w346:string)  [unwired: 14 in]
      }
      frame "Lithography: Run" {
        n126 = Unbundle By Name(w351) -> ("Writing Setpoint"=w358:dbl, "Move Setpoint"=w359:dbl, "Application"=w356:refnum<k7>, "Lithography Data (Conv)"=w361:T8, "Offsets"=w362:cluster{"X":dbl, "Y":dbl}, "Interpolation (um)"=w354:dbl, "Abort Notifier"=w357:refnum<notifier>)
        n127 = Multiply(x=w354, y=1e-06) -> (x*y=w353:dbl)
        n128 = call "Asylum_Driver_LithographyObjects.vi"("Abort Notifier"=w357, "Writing Setpoint"=w358, "Interpolation"=w353, "Move Setpoint"=w359, "error in (no error)"=w366, "Offsets"=w362, "Lithography Data"=w361, "Application"=w356) -> ("error out"=w365:errorcluster, "Application Out"=w350:refnum<k7>)  [unwired: 2 in]
        n129 = Bundle By Name(cluster=w351, "Application"=w350) -> (w352:T7)
        n130 = call <vilib>:"Add State(s) to Queue__JKI_lib_State_Machine.vi"("State(s) in (\"\")"=w364) -> ("States Out"=w363:string)  [unwired: 14 in]
      }
      frame "Lithography: Cleanup" {
        n131 = Unbundle By Name(w369) -> ("Events.Lithography Done"=w368:refnum<user-event>)
        n132 = Generate User Event(user event=w368, event data cluster=TRUE ("event data"), error in=w373) -> (error out=w374:errorcluster)  [unwired: 1 in, 1 out]
        n133 = call <vilib>:"Add State(s) to Queue__JKI_lib_State_Machine.vi"("State(s) in (\"\")"=w372) -> ("States Out"=w371:string)  [unwired: 14 in]
      }
      frame "---------- Asylum ----------" {
        # "Asylum Microscope Functions"
        n134 = call <vilib>:"Add State(s) to Queue__JKI_lib_State_Machine.vi"("State(s) in (\"\")"=w378) -> ("States Out"=w377:string)  [unwired: 14 in]
      }
      frame "Asylum: Close Reference" {
        # "Clear error about reference on Debug Mode"
        # "Asylum Microscope Functions"
        n135 = Unbundle By Name(w382) -> ("Application"=w384:refnum<k7>, "Debug?"=w380:bool)
        n136 = call <userlib>:"Igor_CloseRefnum.vi"("error in (no error)"=w390, "Application"=w384) -> ("error out"=w389:errorcluster)  [unwired: 9 in]
        n137 = case shown="True" w380 {
          tunnel: w389 -> [w391 w394]
          tunnel: [w391 w393] -> w388
          frame False {
          }
          frame True {
            n138 = call <vilib>:"Clear Errors.vi"("error in (no error)"=w394, "specific error code to clear (0: all)"=1045) -> ("error out"=w393:errorcluster)  [unwired: 4 in, 1 out]
          }
        }
        n139 = Bundle By Name(cluster=w382, "Application"=refnum<k7> refnum) -> (w383:T7)
        n140 = call <vilib>:"Add State(s) to Queue__JKI_lib_State_Machine.vi"("State(s) in (\"\")"=w387) -> ("States Out"=w386:string)  [unwired: 14 in]
      }
      frame "Asylum: Open Reference" {
        # "Asylum Microscope Functions"
        n141 = Unbundle By Name(w396) -> ("Debug?"=w395:bool)
        n142 = call <userlib>:"Igor_OpenRefnum.vi"("error in (no error)"=w402, "Debug Mode? (F)"=w395) -> ("error out"=w403:errorcluster, "Application out"=w397:refnum<k7>)  [unwired: 8 in]
        n143 = Bundle By Name(cluster=w396, "Application"=w397) -> (w398:T7)
        n144 = call <vilib>:"Add State(s) to Queue__JKI_lib_State_Machine.vi"("State(s) in (\"\")"=w401) -> ("States Out"=w400:string)  [unwired: 14 in]
      }
      frame "---------- Config ----------" {
        # "Asylum Microscope Functions"
        n145 = Unbundle By Name(w405) -> ("Configuration"=w404:refnum<class "Configuration.lvclass">)
        n146 = Bundle By Name(cluster=w405, "Configuration"=w404) -> (w406:T7)
        n147 = call <vilib>:"Add State(s) to Queue__JKI_lib_State_Machine.vi"("State(s) in (\"\")"=w409) -> ("States Out"=w408:string)  [unwired: 14 in]
      }
      frame "Config: Write" {
        # "Asylum Microscope Functions"
        n148 = Unbundle By Name(w422) -> ("Configuration"=w421:refnum<class "Configuration.lvclass">, "Move Setpoint"=w418:dbl, "Amplifier"=w417:dbl, "Writing Setpoint"=w416:dbl, "Interpolation (um)"=w415:dbl, "Debug?"=w411:bool)
        n149 = Bundle By Name(cluster=T5 {"Move Setpoint"=0.0, "Amplifier"=0.0, "Writing Setpoint"=0.0, "Interpolation"=0.0, "Debug"=TRUE} ("Asylum Config"), "Move Setpoint"=w418, "Amplifier"=w417, "Writing Setpoint"=w416, "Interpolation"=w415, "Debug"=w411) -> (w414:T5)
        n150 = call <userlib>:"Write Configuration.vi"("error in (no error)"=w412, "Variant"=w414, "Configuration in"=w421) -> ("error out"=w413:errorcluster, "Configuration out"=w420:refnum<class "Configuration.lvclass">)  [unwired: 7 in]
        n151 = Bundle By Name(cluster=w422, "Configuration"=w420) -> (w423:T7)
        n152 = call <vilib>:"Add State(s) to Queue__JKI_lib_State_Machine.vi"("State(s) in (\"\")"=w426) -> ("States Out"=w425:string)  [unwired: 14 in]
      }
      frame "Config: Read" {
        w436 = T5 {"Move Setpoint"=0.0, "Amplifier"=0.0, "Writing Setpoint"=0.0, "Interpolation"=0.0, "Debug"=FALSE} ("Asylum Config")
        # "Asylum Microscope Functions"
        n153 = Unbundle By Name(w440) -> ("Configuration"=w439:refnum<class "Configuration.lvclass">)
        n154 = call <userlib>:"Read Configuration.vi"("INI Fomatted Cluster Type"=w436, "error in (no error)"=w433, "Configuration in"=w439) -> ("error out"=w435:errorcluster, "Configuration"=w437:variant, "Configuration out"=w438:refnum<class "Configuration.lvclass">)  [unwired: 6 in]
        n155 = Variant To Data(error in=w435, type=w436, Variant=w437) -> (data=w432:T5, error out=w434:errorcluster)
        n156 = Unbundle By Name(w432) -> ("Writing Setpoint"=w427:dbl, "Move Setpoint"=w428:dbl, "Amplifier"=w429:dbl, "Interpolation"=w430:dbl, "Debug"=w431:bool)
        "Debug Mode?" <- w431
        n157 = local write "Writing Setpoint"(w427) -> ()
        n158 = local write "Move Setpoint"(w428) -> ()
        n159 = local write "Amplifier"(w429) -> ()
        n160 = local write "Interpolation (um)"(w430) -> ()
        n161 = Bundle By Name(cluster=w440, "Configuration"=w438, "Writing Setpoint"=w427, "Move Setpoint"=w428, "Amplifier"=w429, "Interpolation (um)"=w430, "Debug?"=w431) -> (w441:T7)
        n162 = call <vilib>:"Add State(s) to Queue__JKI_lib_State_Machine.vi"("State(s) in (\"\")"=w444) -> ("States Out"=w443:string)  [unwired: 14 in]
      }
      frame "Config: Initialize" {
        # "Asylum Microscope Functions"
        n163 = Unbundle By Name(w451) -> ("Configuration"=w450:refnum<class "Configuration.lvclass">)
        n164 = call "Base INI Folder Path.vi"() -> ("Base Path"=w448:path)  [unwired: 11 in]
        n165 = call <userlib>:"Write Path.vi"("error in (no error)"=w445, "Filename [Configuration.ini]"="Asylum.ini" ("File (Configuration.ini)"), "Path"=w448, "Configuration in"=w450) -> ("error out"=w446:errorcluster, "Configuration out"=w449:refnum<class "Configuration.lvclass">)  [unwired: 6 in]
        n166 = Bundle By Name(cluster=w451, "Configuration"=w449) -> (w452:T7)
        n167 = call <vilib>:"Add State(s) to Queue__JKI_lib_State_Machine.vi"("State(s) in (\"\")"=w455) -> ("States Out"=w454:string)  [unwired: 14 in]
      }
    }
  }
